vi "Property Tree Set Value_Reorder Items.vi"(8 "Error In":errorcluster, 9 "Tag Selected":string[](array[string]), 10 "Active Tree":refnum<vi>, 11 "All Tree Refs":refnum<vi>[](array[refnum])) -> (0 "Error Out":errorcluster)   [LabVIEW 2023]
doc: "Toggle has already happened, so here we determine if row is selecgted and deal with updating the tree value"
panel:
  out "exe time (ms)":u32
  out "Row Selected":bool
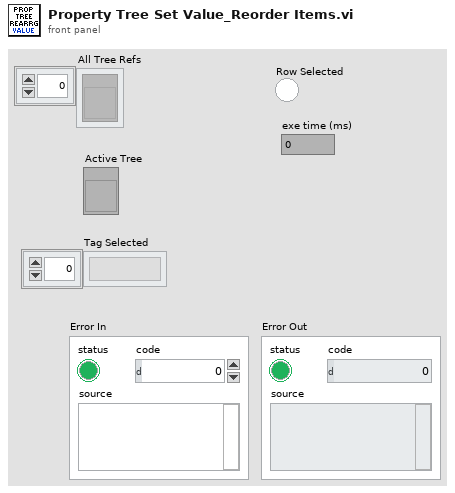
[diagram p1: front panel]
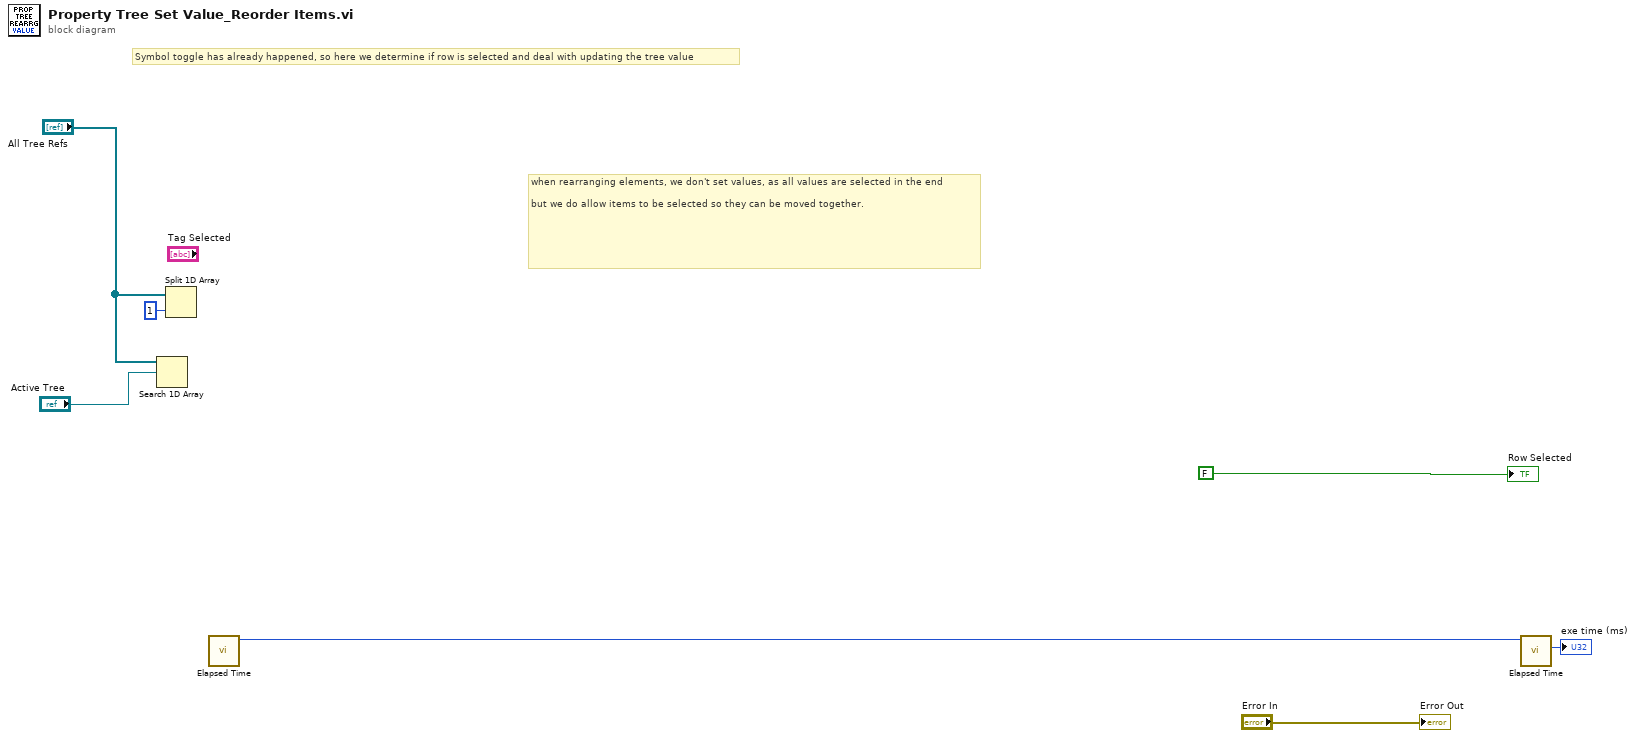
[diagram p0: block diagram]
diagram:
  # "when rearranging elements, we don't set values, as all values are selected in the end\n\nbut we do allow items to be selected so they can be moved together."
  # "Symbol toggle has already happened, so here we determine if row is selected and deal with updating the tree value"
  n1 = Search 1D Array(1D array="All Tree Refs", element="Active Tree") -> ()  [unwired: 1 in, 1 out]
  n2 = Split 1D Array(array="All Tree Refs", index=1) -> ()  [unwired: 2 out]
  n3 = call "Elapsed Time.vi"() -> ("millisecond timer value"=w3:u32)  [unwired: 7 in, 4 out]
  n4 = call "Elapsed Time.vi"("past time"=w3) -> ("elapsed time (ms)"=→"exe time (ms)":u32)  [unwired: 6 in, 4 out]
  "Row Selected" <- FALSE
  "Error Out" <- "Error In"
